vi "Read logFilePath.vi"(11 "Logger in":refnum<class "Log.lvclass">) -> (2 "logFilePath":path, 3 "Logger out":refnum<class "Log.lvclass">)   [LabVIEW 2013, in "Log.lvclass"]
uses:
  Log.lvclass
  Log.lvclass/Log.ctl
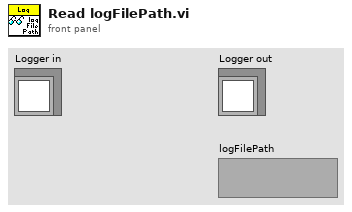
[diagram p1: front panel]
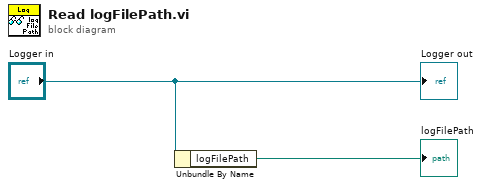
[diagram p0: block diagram]
diagram:
  n1 = Unbundle By Name("Logger in") -> ("logFilePath"=→"logFilePath":path)
  "Logger out" <- "Logger in"
